vi "Read Packet.vi"(0 "comm interface in":refnum<class "Pixy Com.lvclass">, 5 "expected type":u8, 11 "error in":errorcluster) -> (4 "comm interface out":refnum<class "Pixy Com.lvclass">, 6 "type":u8, 8 "received":u8[](array[numeric]), 15 "error out":errorcluster)   [LabVIEW 2018, in "Pixy2.lvlib"]
uses:
  Pixy2.lvlib
  Interface/Pixy Com.lvclass
panel:
  out "length":u8
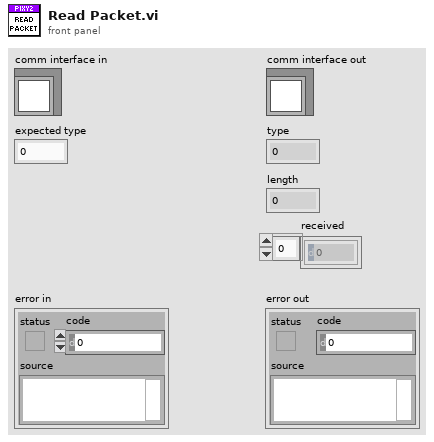
[diagram p1: front panel]
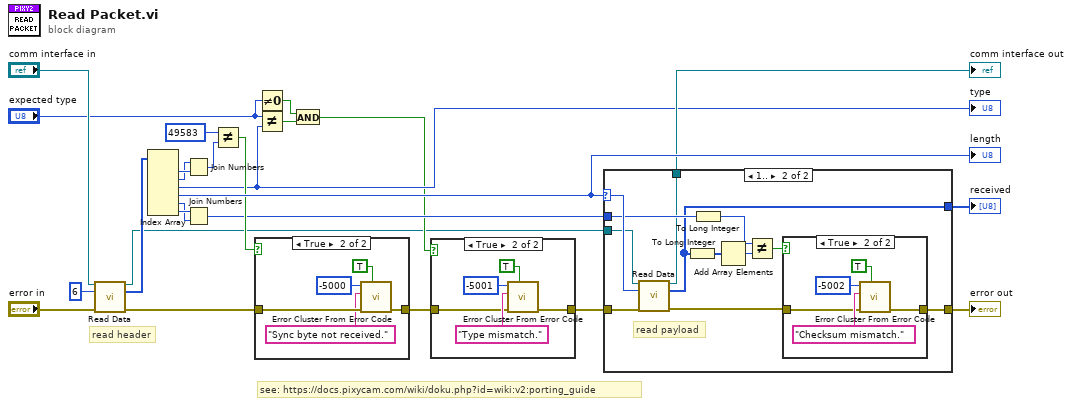
[diagram p0: block diagram]
diagram:
  # "read header"
  # "see: https://docs.pixycam.com/wiki/doku.php?id=wiki:v2:porting_guide"
  n1 = call-dynamic "Read Data.vi"("comm interface in"="comm interface in", "bytes to read"=6, "error in"="error in") -> ("comm interface out"=w1:refnum<class "Pixy Com.lvclass">, "data"=w22:u8[], "error out"=w21:errorcluster)  [unwired: 10 in]
  n2 = Index Array(array=w22) -> (element #1=w20:u8, element #2=w19:u8, element #3=w6:u8, element #4=w16:u8, element #5=w17:u8, element #6=w18:u8)  [unwired: 6 in]
  "type" <- w6
  "length" <- w16
  n3 = Join Numbers(hi=w19, lo=w20) -> ((hi.lo)=w14:u16)
  n4 = Join Numbers(hi=w18, lo=w17) -> ((hi.lo)=w12:u16)
  n5 = Not Equal?(x=u16 49583 ("(hi.lo)"), y=w14) -> (x != y?=w13:bool)
  n6 = case shown="True" w13 {
    tunnel: w21 -> [w26 w31]
    tunnel: [w26 w30] -> w8
    frame False {
    }
    frame True {
      n7 = call <vilib>:"Error Cluster From Error Code.vi"("show call chain? (False)"=TRUE, "error in (no error)"=w31, "error message (\"\")"="Sync byte not received." ("error message (\"\")"), "error code (0)"=-5000) -> ("error out"=w30:errorcluster)  [unwired: 5 in]
    }
  }
  n8 = Not Equal To 0?(x="expected type") -> (x != 0?=w3:bool)
  n9 = Not Equal?(x="expected type", y=w6) -> (x != y?=w4:bool)
  n10 = And(x=w3, y=w4) -> (x .and. y?=w2:bool)
  n11 = case shown="True" w2 {
    tunnel: w8 -> [w32 w34]
    tunnel: [w32 w33] -> w7
    frame False {
    }
    frame True {
      n12 = call <vilib>:"Error Cluster From Error Code.vi"("show call chain? (False)"=TRUE, "error in (no error)"=w34, "error message (\"\")"="Type mismatch." ("error message (\"\")"), "error code (0)"=-5001) -> ("error out"=w33:errorcluster)  [unwired: 5 in]
    }
  }
  n13 = case shown="1.." w16 {
    selector: w16 -> [_ w51]
    tunnel: w12 -> [_ w48]
    tunnel: [w38 w46] -> w11
    tunnel: [w39 w44] -> w10
    tunnel: [_ w43] -> w9
    tunnel: w7 -> [w38 w41]
    tunnel: w1 -> [w39 w40]
    frame ..0 {
    }
    frame 1.. {
      # "read payload"
      n14 = call-dynamic "Read Data.vi"("comm interface in"=w40, "bytes to read"=w51, "error in"=w41) -> ("comm interface out"=w44:refnum<class "Pixy Com.lvclass">, "data"=w43:u8[], "error out"=w42:errorcluster)  [unwired: 10 in]
      n15 = To Long Integer(number=w43) -> (32bit integer=w49:i32[])
      n16 = To Long Integer(number=w48) -> (32bit integer=w47:i32)
      n17 = Add Array Elements(numeric array=w49) -> (sum=w50:i32)
      n18 = Not Equal?(x=w47, y=w50) -> (x != y?=w45:bool)
      n19 = case shown="True" w45 {
        tunnel: w42 -> [w52 w54]
        tunnel: [w52 w53] -> w46
        frame False {
        }
        frame True {
          n20 = call <vilib>:"Error Cluster From Error Code.vi"("show call chain? (False)"=TRUE, "error in (no error)"=w54, "error message (\"\")"="Checksum mismatch." ("error message (\"\")"), "error code (0)"=-5002) -> ("error out"=w53:errorcluster)  [unwired: 5 in]
        }
      }
    }
  }
  "received" <- w9
  "comm interface out" <- w10
  "error out" <- w11
